vi "SP SP - Get current VI name.vi"(8 "error in (no error)":errorcluster, 11 "JSON string":string) -> (0 "error out":errorcluster, 3 "value":string)   [LabVIEW 2020, in "ui-testing.lvlib"]
doc: "copyright: Thomas Zilliox©"
uses:
  ui-testing.lvlib
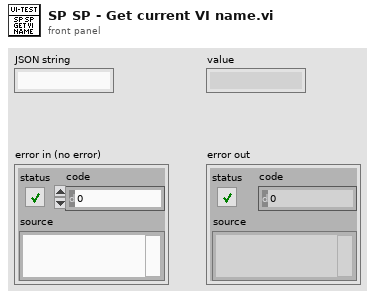
[diagram p1: front panel]
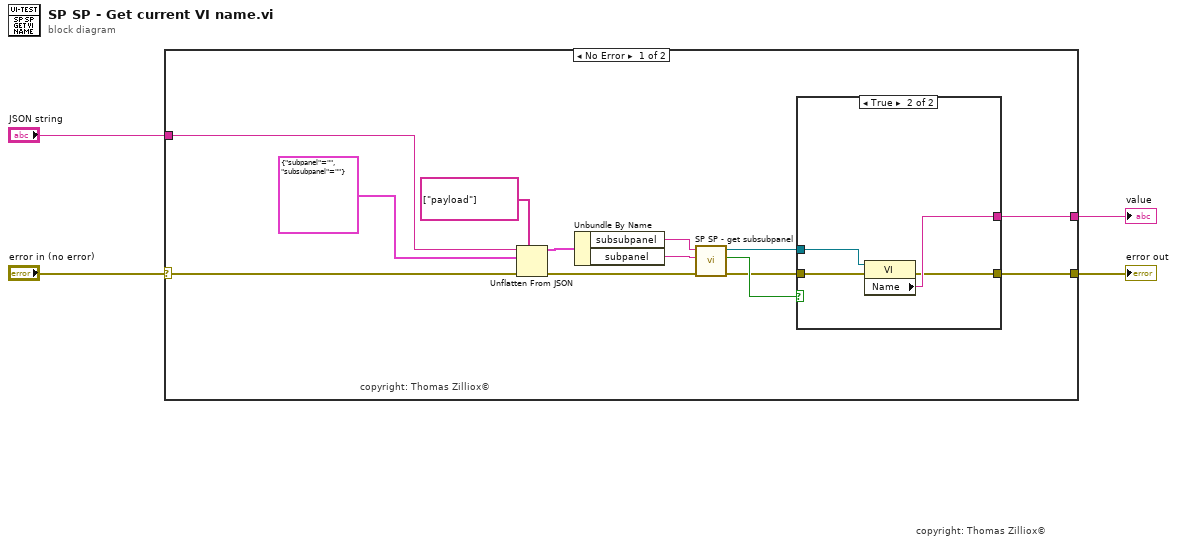
[diagram p0: block diagram]
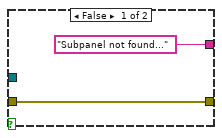
[diagram p2: hidden frame]
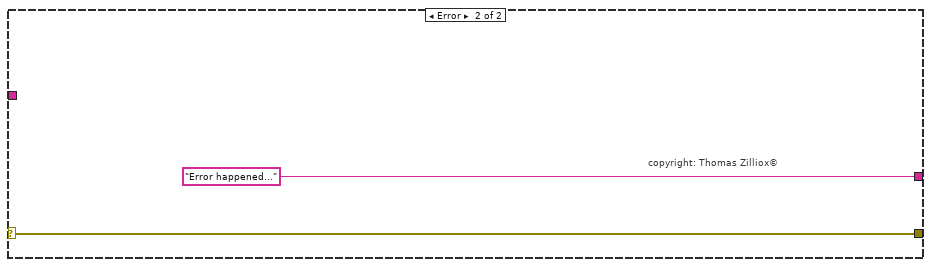
[diagram p3: hidden frame]
diagram:
  # "copyright: Thomas Zilliox©"
  n1 = case shown="No Error" "error in (no error)" {
    selector: "error in (no error)" -> [w10 w25]
    tunnel: "JSON string" -> [w9 _]
    tunnel: [w17 w25] -> w3
    tunnel: [w16 "Error happened..."] -> w1
    frame No Error {
      # "copyright: Thomas Zilliox©"
      n2 = Unflatten From JSON(path=string[] ["payload"], JSON string=w9, type and defaults=cluster{"subpanel":string, "subsubpanel":string} {"subpanel"="", "subsubpanel"=""}, error in (no error)=w10) -> (value=w7:cluster{"subpanel":string, "subsubpanel":string}, error out=w8:errorcluster)  [unwired: 3 in]
      n3 = Unbundle By Name(w7) -> ("subsubpanel"=w5:string, "subpanel"=w6:string)
      n4 = call "SP SP - get subsubpanel.vi"("error in (no error)"=w8, "subpanel"=w6, "subsubpanel"=w5) -> ("error out"=w13:errorcluster, "SubSubPanel found"=w15:bool, "SubSubPanel VI"=w14:refnum<vi>)  [unwired: 5 in, 1 out]
      n5 = case shown="True" w15 {
        tunnel: w13 -> [w18 w23]
        tunnel: [w18 w21] -> w17
        tunnel: ["Subpanel not found..." ("Name") w22] -> w16
        tunnel: w14 -> [_ w20]
        frame False {
        }
        frame True {
          n6 = property class="VI"(reference=w20, error in=w23) -> (error out=w21:errorcluster, "Name"=w22:string)  [unwired: 1 out]
        }
      }
    }
    frame Error {
      # "copyright: Thomas Zilliox©"
    }
  }
  "error out" <- w3
  "value" <- w1
